vi "Ver 1.5.vi"() -> ()   [LabVIEW 2015]
uses:
  <instrlib>/Keithley 622x LV 2009/Configure/Source/Typedefs/KE622x -- Current Range.ctl
  <instrlib>/Keithley 622x LV 2009/Configure/Source/Typedefs/KE622x -- Current Ranges.ctl
  <instrlib>/Keithley 622x LV 2009/Typedefs/KE622x -- On Off Control.ctl
  <instrlib>/Keithley 622x LV 2009/Configure/Source/Typedefs/KE622x -- Voltage Limit.ctl
  <instrlib>/Keithley 622x LV 2009/Utility/Typedefs/KE622x -- Instrument Type.ctl
  <instrlib>/Keithley 2000/Public/Configure/Configure DC Volts.vi
  <userlib>/LV-Link3/PolySubVIs/DtCreateAinChan.vi
  <userlib>/LV-Link3/PolySubVIs/DtOLReadSingle.vi
  <instrlib>/Keithley 2000/Keithley 2000.lvlib
  <instrlib>/Keithley 622x LV 2009/Keithley 622x.lvlib
panel:
  out "DAQ":dbl format="%#_13g"
  out "2000":dbl format="%#_13g"
  in  "Device":string(combo)
  in  "Channels":string="0"
  in  "Number \nof points":i32
  in  "Folder\nprename":string
  out "XY Graph":cluster{u32[], dbl[]}[](graph)
  out "T0":u32
  out "LIMIT":bool
  out "LIMIT":bool
  out "Error Code":string
  in  "Comments":string
  out "file":refnum<file>
  out "2000":refnum<visa-resource-name>
  out "6221":refnum<visa-resource-name>
  out "Step  (A)":dbl=5e-05 format="%#_3p"
  in  "Stop\ncurrent (A)":dbl=0.002 format="%#_6p"
  in  "Start \ncurrent (A)":dbl=0.001 format="%#_6p"
  in  "Check For SCPI Errors? (T)":bool=TRUE
  out "Interlock Tripped?":bool
  out "Compliance?":bool
  in  "Turn Off Output \nIf Compliance?":bool=TRUE
  in  "Turning ON/OFF\ncurrent output":T1=enum."On"
  in  "Range Selection":T2={"Auto Range?"=TRUE, "Man / Selected\nRange"=enum."2nA"}
  # "FILE CONFIGURATION"
  # "ADMIN PANEL"
  # "READINGS"
  # "KEITHLEY 6221 CONFIGURATION (ADMIN ONLY)"
  # "KEITHLEY DAQ CONFIGURATION (ADMIN ONLY)"
  # "I don't know what the hell it is,\njust don't touch it"
  # "START, STOP, STEP, CONFIGURATION"
  # "IF ON"
  # "Compliance = Limiting output voltage\nThis switch determines if we want to switch \noff the current output if wee exceed compliance"
  # "There is a safe switch at \nthe back of the instrument \nThis indicator shows if it is on"
  # "You have hit a damn jackpot \nby exceeding the limited voltage\nCongrats"
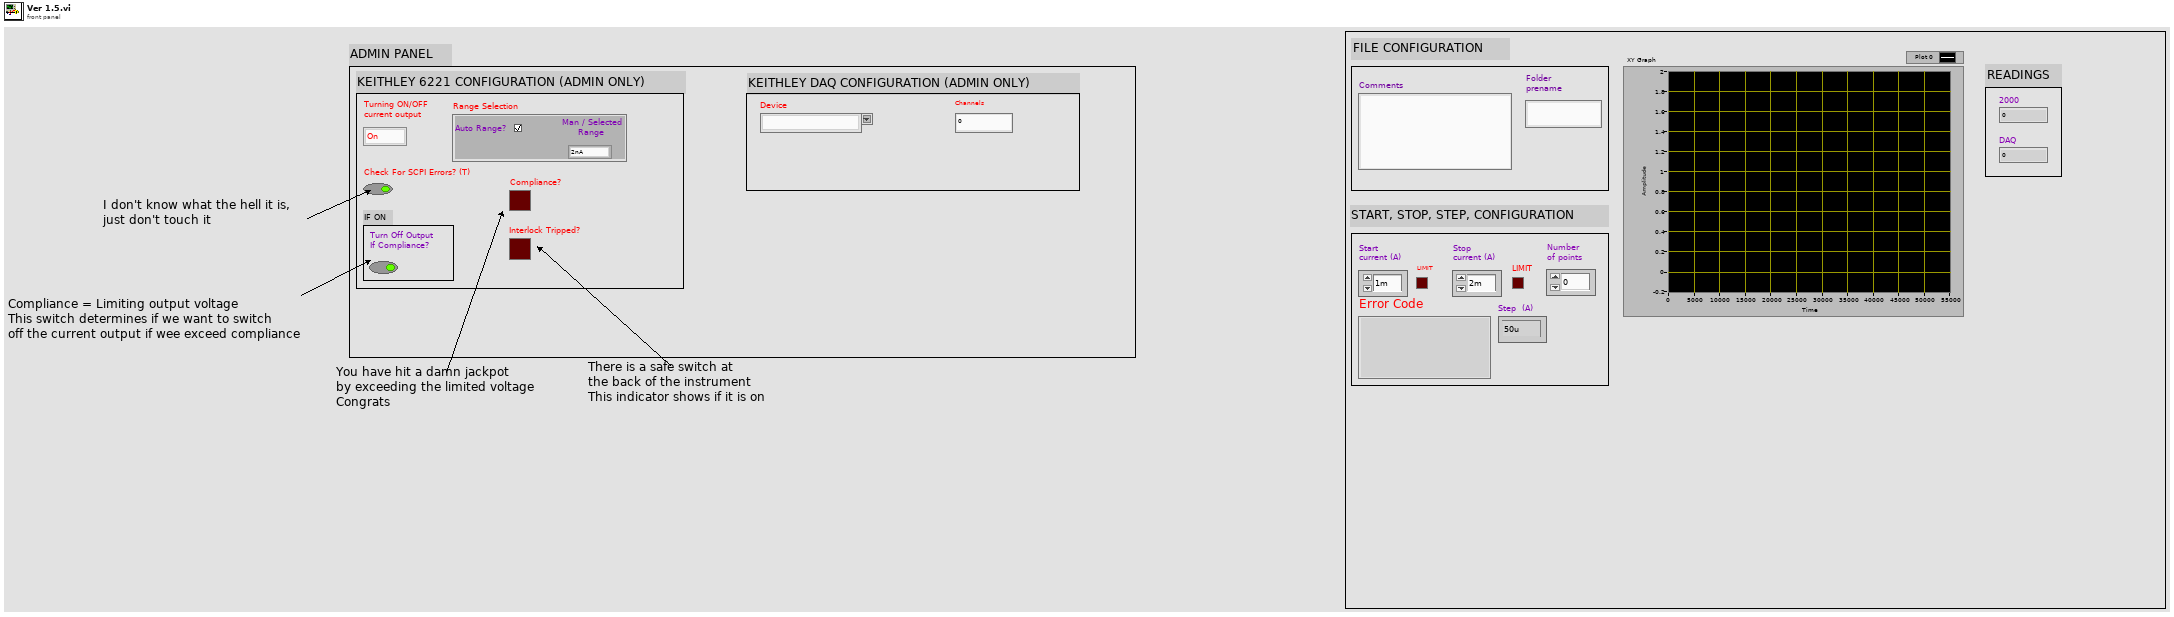
[diagram p1: front panel]
types:
  T1 = typedef "Keithley 622x.lvlib/KE622x -- On Off Control.ctl" = enum16{"Off", "On"}
  T2 = typedef "Keithley 622x.lvlib/KE622x -- Current Range.ctl" = cluster{"Auto Range?":bool, "Man / Selected\nRange":T3}
  T3 = typedef "Keithley 622x.lvlib/KE622x -- Current Ranges.ctl" = enum16{"2nA", "20nA", "200nA", "2uA", "20uA", "200uA", "2mA", "20mA", "100mA"}
  T4 = typedef "Keithley 622x.lvlib/KE622x -- Voltage Limit.ctl" = dbl
  T5 = typedef "Keithley 622x.lvlib/KE622x -- Instrument Type.ctl" = enum16{"KE6220", "KE6221"}
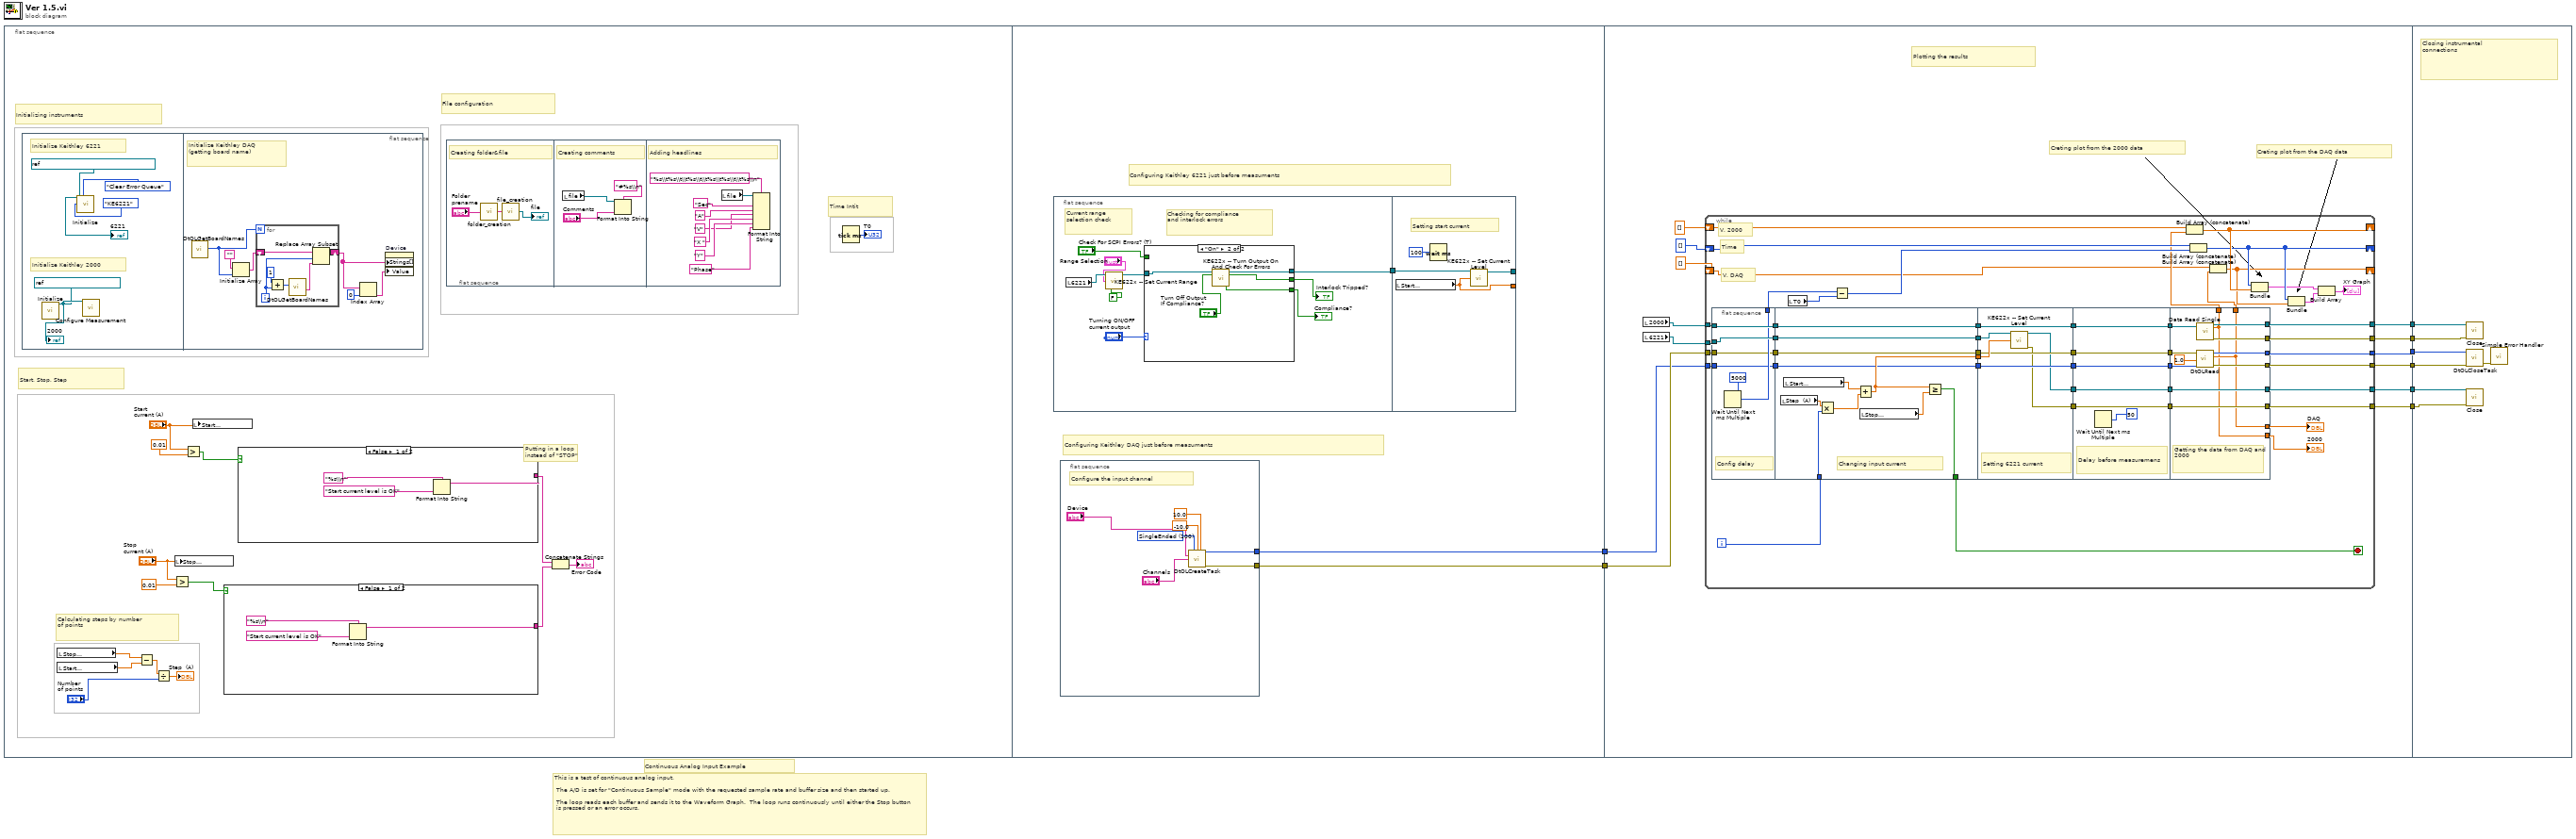
[diagram p0: block diagram]
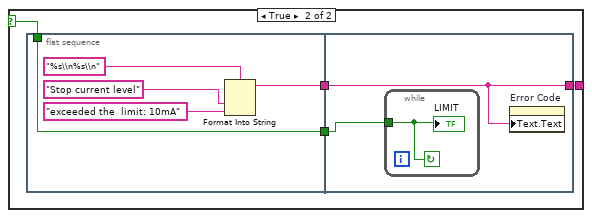
[diagram p2: hidden frame]
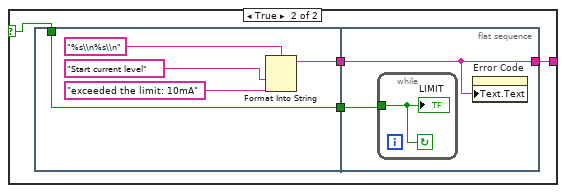
[diagram p3: hidden frame]
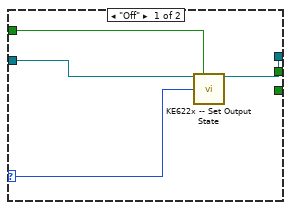
[diagram p4: hidden frame]
diagram:
  # "Continuous Analog Input Example"
  # "This is a test of continuous analog input. \n\n The A/D is set for \"Continuous Sample\" mode with the requested sample rate and buffer size and then started up.\n\n The loop reads each buffer and sends it to the Waveform Graph.  The loop runs continuously until either the Stop button\n is pressed or an error occurs."
  n1 = flat-sequence {
    tunnel: [w87] -> w8
    tunnel: [w86] -> w7
    tunnel: w8 -> [w127]
    tunnel: w7 -> [w128]
    tunnel: [w126] -> w6
    tunnel: [w124] -> w5
    tunnel: [w123] -> w4
    tunnel: [w122] -> w3
    tunnel: [w121] -> w2
    tunnel: [w120] -> w1
    tunnel: w6 -> [w225]
    tunnel: w5 -> [w224]
    tunnel: w4 -> [w223]
    tunnel: w3 -> [w222]
    tunnel: w2 -> [w221]
    tunnel: w1 -> [w220]
    frame #0 {
      # "Calculating steps by number\nof points"
      # "Time Intit"
      # "Putting in a loop \ninstead of \"STOP\""
      # "Start, Stop, Step"
      # "Initializing instruments"
      # "File configuration"
      n2 = flat-sequence {
        frame #0 {
          # "Initialize Keithley 2000"
          # "Initialize Keithley 6221"
          n3 = call <instrlib>:"Initialize.vi"("VISA resource name"=refnum<visa-resource-name> "KEITHLEY_MULTIMETER") -> ("VISA resource name out"=w25:refnum<visa-resource-name>)  [unwired: 17 in, 1 out]
          "2000" <- w25
          n4 = call <instrlib>:"Initialize.vi"("VISA resource name"=refnum<visa-resource-name> "KEITHLEY_DC_AC_CURRENT_SOURCE", "Error Queue Option"=enum16{"Clear Error Queue", "Error Query"}."Clear Error Queue", "Instrument Type"=KE622x_--_Instrument_Type."KE6221") -> ("VISA resource name out"=→"6221":refnum<visa-resource-name>)  [unwired: 11 in, 1 out]
          n5 = call-poly <instrlib>:"Configure Measurement.vi"("VISA resource name"=w25) -> ()  [unwired: 17 in, 2 out]
        }
        frame #1 {
          # "Initialize Keithley DAQ \n(getting board name)"
          n6 = call <userlib>:"DtOLGetBoardNames.vi"() -> ("Number of boards"=w30:u32)  [unwired: 9 in, 2 out]
          n7 = Initialize Array("", w30) -> (w32:string[])
          n8 = for {
            N: w30 -> [_]
            shift-right: [w38] -> w35
            shift-left: w32 -> [w39]
            i -> [w37]
            n9 = Add(x=1, y=w37) -> (x+y=w41:i32)
            n10 = call <userlib>:"DtOLGetBoardNames.vi"("Select Board"=w41) -> ("Board Name"=w36:string)  [unwired: 8 in, 2 out]
            n11 = Replace Array Subset(array=w39, new element=w36, index=w37) -> (w38:string[])
          }
          n12 = Index Array(array=w35, index=0) -> (element=w34:string)
          n13 = property on="Device" class="CmbBox"("Strings[]"=w35, "Value"=w34) -> ()  [unwired: 2 in, 2 out]
        }
      }
      n14 = local read "Stop\ncurrent (A)"() -> (w12:dbl)
      n15 = local read "Start \ncurrent (A)"() -> (w11:dbl)
      n16 = Subtract(x=w12, y=w11) -> (x-y=w9:dbl)
      n17 = Divide(x=w9, y="Number \nof points") -> (x/y=→"Step  (A)":dbl)
      n18 = Greater?(x="Stop\ncurrent (A)", y=T4 0.01) -> (0:w18:bool)
      n19 = local write "Stop\ncurrent (A)"("Stop\ncurrent (A)") -> ()
      n20 = Greater?(x="Start \ncurrent (A)", y=T4 0.01) -> (0:w19:bool)
      n21 = local write "Start \ncurrent (A)"("Start \ncurrent (A)") -> ()
      n22 = case shown="False" w18 {
        selector: w18 -> [_ w45]
        tunnel: [w42 w48] -> w16
        frame False {
          n23 = Format Into String(format string="%s\\n", "Start current level is OK" ("false string")) -> (resulting string=w42:string)  [unwired: 2 in, 1 out]
        }
        frame True {
          n24 = flat-sequence {
            tunnel: [w50] -> w47
            tunnel: [w49] -> w46
            tunnel: w45 -> [w49]
            tunnel: [w54] -> w48
            tunnel: w47 -> [w54]
            tunnel: w46 -> [w55]
            frame #0 {
              n25 = Format Into String(format string="%s\\n%s\\n", "Stop current level" ("String"), "exceeded the  limit: 10mA" ("input 2")) -> (resulting string=w50:string)  [unwired: 2 in, 1 out]
            }
            frame #1 {
              n26 = while {
                tunnel: w55 -> [w56]
                stop <- w56 continue-if-true
                "LIMIT" <- w56
              }
              n27 = property on="Error Code" class="Str"("Text.Text"=w54) -> ()  [unwired: 2 in, 2 out]
            }
          }
        }
      }
      n28 = case shown="False" w19 {
        selector: w19 -> [_ w61]
        tunnel: [w57 w63] -> w17
        frame False {
          n29 = Format Into String(format string="%s\\n", "Start current level is OK" ("false string")) -> (resulting string=w57:string)  [unwired: 2 in, 1 out]
        }
        frame True {
          n30 = flat-sequence {
            tunnel: [w65] -> w62
            tunnel: w61 -> [w64]
            tunnel: [w64] -> w60
            tunnel: [w69] -> w63
            tunnel: w62 -> [w69]
            tunnel: w60 -> [w70]
            frame #0 {
              n31 = Format Into String(format string="%s\\n%s\\n", "Start current level" ("String"), "exceeded the limit: 10mA" ("input 2")) -> (resulting string=w65:string)  [unwired: 2 in, 1 out]
            }
            frame #1 {
              n32 = while {
                tunnel: w70 -> [w71]
                stop <- w71 continue-if-true
                "LIMIT" <- w71
              }
              n33 = property on="Error Code" class="Str"("Text.Text"=w69) -> ()  [unwired: 2 in, 2 out]
            }
          }
        }
      }
      n34 = flat-sequence {
        frame #0 {
          # "Creating folder&file"
          n35 = call "folder_creation.vi"("Name"="Folder\nprename") -> ("String"=w73:string)
          n36 = call "file_creation.vi"("String"=w73) -> ("refnum out"=→"file":refnum<file>)
        }
        frame #1 {
          # "Creating comments"
          n37 = local read "file"() -> (w75:refnum<file>)
          n38 = Format Into String(format string="#%s\\n", initial string=w75, "Comments") -> ()  [unwired: 1 in, 2 out]
        }
        frame #2 {
          # "Adding headlines"
          n39 = local read "file"() -> (w85:refnum<file>)
          n40 = Format Into String(format string="%s\\t%s\\t\\t%s\\t\\t%s\\t%s\\t\\t%s\\n", initial string=w85, "Sec" ("input 1"), "A" ("input 2"), "V" ("input 3"), "X " ("input 3"), "Y" ("input 3"), "Phase" ("input 3")) -> ()  [unwired: 1 in, 2 out]
        }
      }
      n41 = Concatenate Strings(w17, w16) -> (→"Error Code":string)
      n42 = Tick Count (ms)() -> (millisecond timer value=→"T0":u32)
    }
    frame #1 {
      # "Configuring Keithley DAQ just before measuments"
      # "Configuring Keithley 6221 just before measuments"
      n43 = flat-sequence {
        tunnel: [w96] -> w88
        tunnel: [w114] -> _
        tunnel: [w116] -> _
        tunnel: w88 -> [w115]
        frame #0 {
          # "Current range \nselection check"
          # "Checking for compliance\nand interlock errors"
          n44 = local read "6221"() -> (w99:refnum<visa-resource-name>)
          n45 = call <instrlib>:"KE622x -- Set Current Range.vi"("Resource In"=w99, "Current Range In"="Range Selection", "Read Back Set Values? (T)"=FALSE) -> ("Resource Out (dupl)"=w104:refnum<visa-resource-name>)  [unwired: 10 in, 2 out]
          n46 = case shown="\"On\"" "Turning ON/OFF\ncurrent output" {
            selector: "Turning ON/OFF\ncurrent output" -> [w108 _]
            tunnel: [_ w112] -> w102
            tunnel: [_ w111] -> w103
            tunnel: "Check For SCPI Errors? (T)" -> [w107 _]
            tunnel: w104 -> [w105 w110]
            tunnel: [w106 w109] -> w96
            frame "Off" {
              n47 = call <instrlib>:"KE622x -- Set Output State.vi"("Resource In"=w105, "Check For SCPI Errors? (T)"=w107, "Output State"=w108) -> ("Resource Out (dupl)"=w106:refnum<visa-resource-name>)  [unwired: 11 in, 1 out]
            }
            frame "On" {
              n48 = call <instrlib>:"KE622x -- Turn Output On And Check For Errors.vi"("Resource In"=w110, "Turn Off Output If Compliance?"="Turn Off Output \nIf Compliance?") -> ("Resource Out (dupl)"=w109:refnum<visa-resource-name>, "Interlock Tripped?"=w112:bool, "Compliance?"=w111:bool)  [unwired: 10 in, 1 out]
            }
          }
          "Interlock Tripped?" <- w102
          "Compliance?" <- w103
        }
        frame #1 {
          # "Setting start current"
          n49 = local read "Start \ncurrent (A)"() -> (w114:dbl)
          n50 = Wait (ms)(milliseconds to wait=u32 100) -> ()  [unwired: 1 out]
          n51 = call <instrlib>:"KE622x -- Set Current Level.vi"("Resource In"=w115, "Current Level (A) In"=w114) -> ("Resource Out (dupl)"=w116:refnum<visa-resource-name>)  [unwired: 12 in, 1 out]
        }
      }
      n52 = flat-sequence {
        tunnel: [w90] -> w87
        tunnel: [w89] -> w86
        frame #0 {
          w94 = 100 items=["SingleEnded"=100, "Differential"=101] ("Channel Type")
          # "Configure the input channel"
          n53 = call-poly <userlib>:"DtOLCreateTask.vi"("Channel Type"=w94, "Range Min"=-10.0, "Range Max"=10.0, "Board Name"="Device", "Channel"="Channels") -> ("Task out"=w90:i32, "error out"=w89:errorcluster)  [unwired: 8 in, 1 out]
        }
      }
    }
    frame #2 {
      # "Plotting the results"
      # "Creting plot from the DAQ data"
      # "Creting plot from the 2000 data"
      n54 = local read "2000"() -> (w119:refnum<visa-resource-name>)
      n55 = local read "6221"() -> (w118:refnum<visa-resource-name>)
      n56 = while {
        shift-right: [w147] -> _
        shift-left: dbl[] [] -> [w177]
        shift-right: [w146] -> _
        shift-left: i32[] [] -> [w176]
        tunnel: w119 -> [w173]
        tunnel: w118 -> [w171]
        tunnel: w128 -> [w154]
        tunnel: w127 -> [w149]
        tunnel: [w160] -> w126
        shift-right: [w145] -> _
        shift-left: dbl[] [] -> [w159]
        tunnel: [w141] -> w124
        tunnel: [w140] -> w123
        tunnel: [w139] -> w122
        tunnel: [w137] -> w121
        tunnel: [w134] -> w120
        i -> [w167]
        stop <- w161 stop-if-true
        # "Time"
        # "V, DAQ"
        # "V, 2000"
        n57 = flat-sequence {
          tunnel: w173 -> [w183]
          tunnel: [w183] -> w172
          tunnel: w171 -> [w182]
          tunnel: [w182] -> w170
          tunnel: [w180] -> w169
          tunnel: [w179] -> w155
          tunnel: w154 -> [w179]
          tunnel: [w178] -> w150
          tunnel: w149 -> [w178]
          tunnel: [w194] -> w166
          tunnel: w172 -> [w194]
          tunnel: w170 -> [w189]
          tunnel: w167 -> [w191]
          tunnel: [w187] -> w161
          tunnel: [w186] -> w164
          tunnel: [w189] -> w163
          tunnel: [w185] -> w156
          tunnel: w155 -> [w185]
          tunnel: [w184] -> w151
          tunnel: w150 -> [w184]
          tunnel: w166 -> [w201]
          tunnel: [w201] -> w165
          tunnel: w164 -> [w200]
          tunnel: w163 -> [w199]
          tunnel: [w198] -> w157
          tunnel: w156 -> [w198]
          tunnel: [w197] -> w152
          tunnel: w151 -> [w197]
          tunnel: [w196] -> w138
          tunnel: [w195] -> w135
          tunnel: w165 -> [w207]
          tunnel: [w207] -> w168
          tunnel: [w205] -> w158
          tunnel: w157 -> [w205]
          tunnel: [w204] -> w153
          tunnel: w152 -> [w204]
          tunnel: w138 -> [w203]
          tunnel: [w203] -> w136
          tunnel: w135 -> [w202]
          tunnel: [w202] -> w133
          tunnel: w168 -> [w219]
          tunnel: [w208] -> w162
          tunnel: [w217] -> w160
          tunnel: w158 -> [w216]
          tunnel: w153 -> [w215]
          tunnel: [w209] -> w148
          tunnel: [w214] -> w141
          tunnel: [w213] -> w140
          tunnel: [w212] -> w139
          tunnel: [w211] -> w137
          tunnel: w136 -> [w211]
          tunnel: [w210] -> w134
          tunnel: w133 -> [w210]
          tunnel: [w209] -> w132
          tunnel: [w208] -> w131
          frame #0 {
            # "Config delay"
            n58 = Wait Until Next ms Multiple(millisecond multiple=u32 5000) -> (millisecond timer value=w180:u32)
          }
          frame #1 {
            # "Changing input current"
            n59 = local read "Step  (A)"() -> (w192:dbl)
            n60 = local read "Start \ncurrent (A)"() -> (w193:dbl)
            n61 = Multiply(x=w192, y=w191) -> (x*y=w190:dbl)
            n62 = Add(x=w193, y=w190) -> (x+y=w186:dbl)
            n63 = local read "Stop\ncurrent (A)"() -> (w188:dbl)
            n64 = Greater Or Equal?(x=w186, y=w188) -> (x >= y?=w187:bool)
          }
          frame #2 {
            # "Setting 6221 current"
            n65 = call <instrlib>:"KE622x -- Set Current Level.vi"("Resource In"=w199, "Current Level (A) In"=w200) -> ("Resource Out (dupl)"=w195:refnum<visa-resource-name>, "error out"=w196:errorcluster)  [unwired: 12 in]
          }
          frame #3 {
            # "Delay before measuremens"
            n66 = Wait Until Next ms Multiple(millisecond multiple=u32 50) -> ()  [unwired: 1 out]
          }
          frame #4 {
            # "Getting the data from DAQ and 2000"
            n67 = call-poly <userlib>:"DtOLRead.vi"("error in (no error)"=w216, "Timeout"=1.0, "Task in"=w215) -> ("error out"=w212:errorcluster, "Data Out"=w209:dbl, "Task out"=w217:i32)  [unwired: 6 in]
            n68 = call <instrlib>:"Data Read Single.vi"("VISA resource name"=w219) -> ("VISA resource name out"=w213:refnum<visa-resource-name>, "Measurement"=w208:dbl, "error out"=w214:errorcluster)  [unwired: 14 in, 2 out]
          }
        }
        n69 = local read "T0"() -> (w175:u32)
        n70 = Subtract(x=w169, y=w175) -> (x-y=w174:u32)
        n71 = Build Array (concatenate)(w177, w162) -> (w147:dbl[])
        n72 = Build Array (concatenate)(w176, w174) -> (w146:u32[])
        n73 = Build Array (concatenate)(w159, w148) -> (w145:dbl[])
        n74 = Bundle(w146, w147) -> (w143:cluster{u32[], dbl[]})  [unwired: 1 in]
        n75 = Bundle(w146, w145) -> (w142:cluster{u32[], dbl[]})  [unwired: 1 in]
        n76 = Build Array(w143, w142) -> (→"XY Graph":cluster{u32[], dbl[]}[])
        "2000" <- w131
        "DAQ" <- w132
      }
    }
    frame #3 {
      # "Closing instrumental \nconnections"
      n77 = call <instrlib>:"Close.vi"("VISA resource name"=w223, "error in (no error)"=w224) -> ()  [unwired: 17 in, 1 out]
      n78 = call <userlib>:"DtOLCloseTask.vi"("Error in"=w222, "Task in"=w225) -> ("Error Out"=w226:errorcluster)  [unwired: 9 in]
      n79 = call <instrlib>:"Close.vi"("VISA resource name"=w220, "error in (no error)"=w221) -> ()  [unwired: 13 in, 1 out]
      n80 = call <vilib>:"Simple Error Handler.vi"("error in (no error)"=w226) -> ()  [unwired: 4 in, 5 out]
    }
  }
